vi "ControlAcceleration.vi"(1 "Max Acceleration (power/s)":dbl, 2 "Raw":dbl) -> (0 "Controlled":dbl)   [LabVIEW 2018]
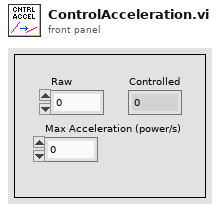
[diagram p1: front panel]
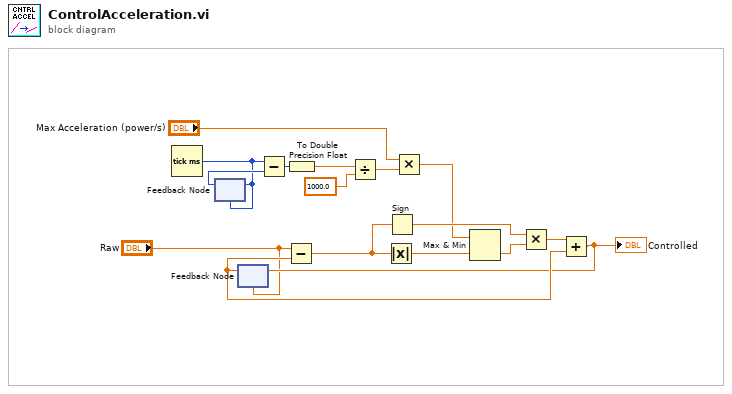
[diagram p0: block diagram]
diagram:
  n1 = Tick Count (ms)() -> (millisecond timer value=w9:u32)
  n2 = feedback-in #1(w9) -> ()
  n3 = feedback #1(w9) -> (w10:u32)
  n4 = feedback #2("Raw") -> (w11:dbl)
  n5 = Subtract(x=w9, y=w10) -> (x-y=w8:u32)
  n6 = Subtract(x="Raw", y=w11) -> (x-y=w16:dbl)
  n7 = To Double Precision Float(number=w8) -> (double precision float=w5:dbl)
  n8 = Divide(x=w5, y=1000.0) -> (x/y=w4:dbl)
  n9 = Absolute Value(x=w16) -> (abs(x)=w15:dbl)
  n10 = Sign(1:w16) -> (0:w14:dbl)
  n11 = Multiply(x="Max Acceleration (power/s)", y=w4) -> (x*y=w7:dbl)
  n12 = Max & Min(x=w7, y=w15) -> (min(x,y)=w13:dbl)  [unwired: 1 out]
  n13 = Multiply(x=w14, y=w13) -> (x*y=w12:dbl)
  n14 = Add(x=w12, y=w11) -> (x+y=w2:dbl)
  "Controlled" <- w2
  n15 = feedback-in #2(w2) -> ()
